vi "Custom User Scripting For New Override VI.vi"(8 "error in":errorcluster, 11 "VI Refnum in":refnum<vi>) -> (0 "error out":errorcluster)   [LabVIEW 2021]
doc: "When \"New >> VI For Override...\" is used to create a VI, this subVI will be invoked if the VI is created successfully after all other work to create the VI has been completed. Users may edit this subVI to add any instructions they wish for customizations of the newly generated VI."
panel:
  # "When \"New >> VI For Override...\" is used to create a VI, this subVI will be invoked if the VI is created successfully after all other work to create the VI has been completed. Users may edit this subVI to add any instructions they wish for customizations of the newly generated VI."
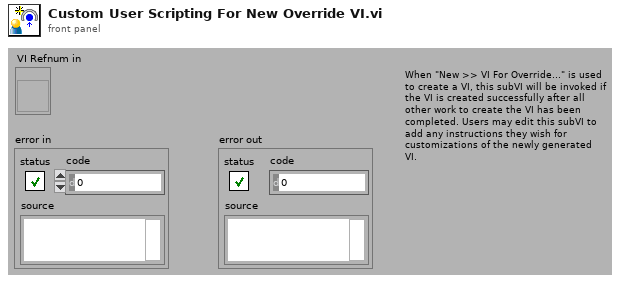
[diagram p1: front panel]
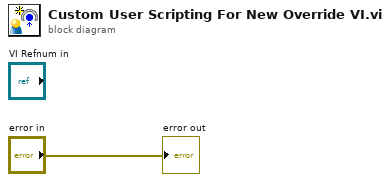
[diagram p0: block diagram]
diagram:
  "error out" <- "error in"
